vi "Detect change of parameters.vi"(10 "AOL_Globals":T1={"Imaging Protocol"=enum."AOL Z-Stack", "Number of POI"=0, "Number of Miniscans"=0, "Number of Trials"=0, "Number of Cycles "=0, "# Averaged Frames"=0, "Laser power (%)"=0, "Pockels"=0.0, "Acquisition Length (sec)"=0.0, "Fill time (us)"=0.0, "POI Dwell time (us)"=0.0, "Miniscan Dwell time per pixel (us)"=0.0, "PMT 1"=0.0, "PMT 2"=0.0, "Back Apperture"=0.0, "Frame Size"=0, "Center Frequency"=0.0, "Field of View"=0.0, "DwellTime (us)"=0.0, "Wavelength (nm)"=0.0, "Zoom"=0.0, "AOL Z"=0.0, "AOL Mode"=enum."Raster", "GridXY"=0.0, "GridZ"=0.0, "TriggerPeriod (sec)"=0.0, "Number of Pixels in Miniscan"=0, "Experiment folder path"=path "", "X centre"=0.0, "Y centre"=0.0, "Angle (degrees)"=0.0, "Plane Mode"=0, "Threshold"=[], "Regenerate Chirps"=FALSE, "Rectangle ROI length (pixels)"=0, "Rectangle ROI height (pixels)"=0, "AOD fill"=0, "Samples Wait after Trigger"=0, "StartUp Delay"=0, "Slip Cycle"=163840, "Add Cycle"=FALSE} {"Plane Mode" items=["XY Plane"]; "Frame Size" items=["100X100"=100, "128X128"=128, "200X200"=200, "256X256"=256, "512X512"=512, "1024x1024"=1024, "2048x2048"=2048]; "Back Apperture" format="%#.6g"; "Pockels" format="%#.6g"; "PMT 2" format="%#.6g"; "PMT 1" format="%#.6g"; "Angle (degrees)" format="%#.6g"; "POI Dwell time (us)" format="%#.6g"}, 11 "ZStack":cluster{"Zstart":dbl, "Zstop":dbl, "Zstep":dbl}) -> (3 "Setup has changed":bool)   [LabVIEW 2013]
uses:
  Typedefs/Controls/AOL_Globals.ctl
  Typedefs/Imaging Protocols enum.ctl
  Typedefs/Frame Size.ctl
  Typedefs/AOL modes.ctl
  Typedefs/Plane Mode.ctl
  Typedefs/Chirps regen checked params.ctl
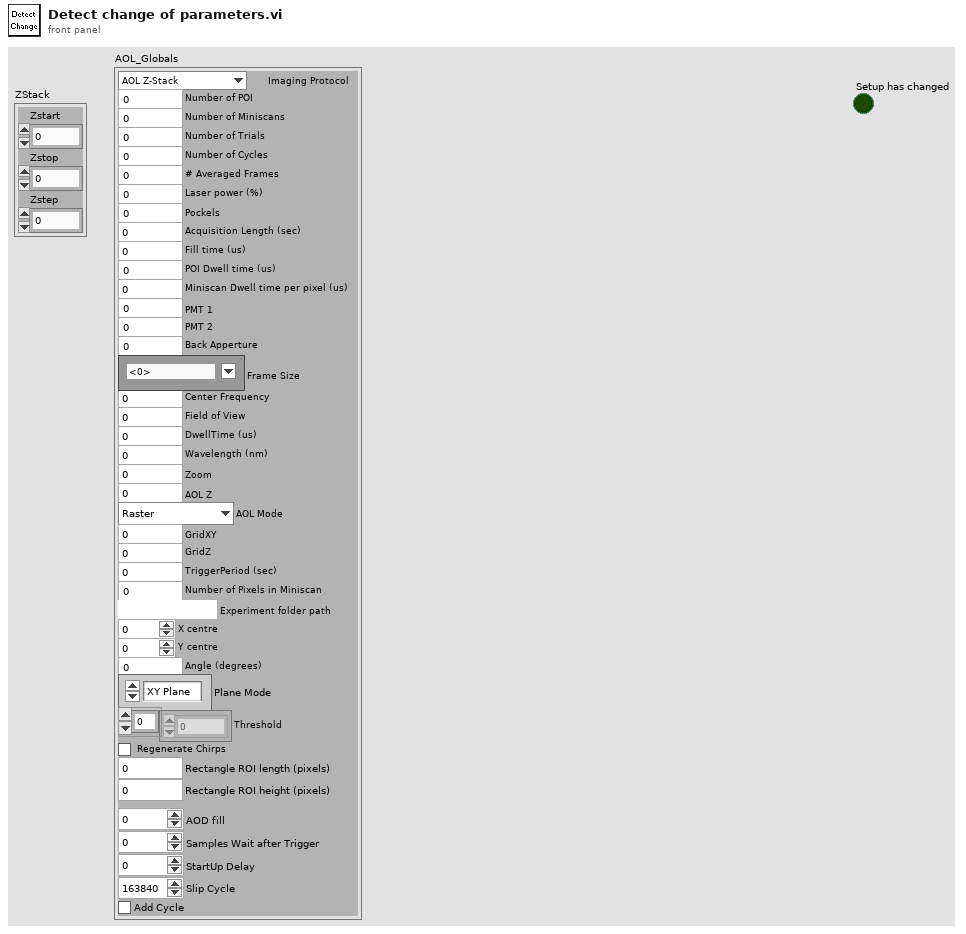
[diagram p1: front panel]
types:
  T1 = typedef "AOL_Globals.ctl" = cluster{"Imaging Protocol":T2, "Number of POI":u16, "Number of Miniscans":u16, "Number of Trials":u16, "Number of Cycles ":u64, "# Averaged Frames":u16, "Laser power (%)":u8, "Pockels":dbl, "Acquisition Length (sec)":dbl, "Fill time (us)":dbl, "POI Dwell time (us)":dbl, "Miniscan Dwell time per pixel (us)":dbl, "PMT 1":dbl, "PMT 2":dbl, "Back Apperture":dbl, "Frame Size":T3, "Center Frequency":dbl, "Field of View":dbl, "DwellTime (us)":dbl, "Wavelength (nm)":dbl, "Zoom":dbl, "AOL Z":dbl, "AOL Mode":T4, "GridXY":dbl, "GridZ":dbl, "TriggerPeriod (sec)":dbl, "Number of Pixels in Miniscan":u16, "Experiment folder path":path, "X centre":dbl, "Y centre":dbl, "Angle (degrees)":dbl, "Plane Mode":T5, "Threshold":u16[], "Regenerate Chirps":bool, "Rectangle ROI length (pixels)":u16, "Rectangle ROI height (pixels)":u16, "AOD fill":u16, "Samples Wait after Trigger":u16, "StartUp Delay":i32, "Slip Cycle":u32, "Add Cycle":bool}
  T2 = typedef "Imaging Protocols enum.ctl" = enum16{"AOL Z-Stack", "Motor Z Stack", "Functional Acquisition", "Single Plane Acquisition", "Volume Acquisition", "Live Imaging", "Live Plane Imaging", "Live Volume Imaging"}
  T3 = typedef "Frame Size.ctl" = u16
  T4 = typedef "AOL modes.ctl" = enum16{"Raster", "Structural", "Pointing", "Mini Scan", "Alignment"}
  T5 = typedef "Plane Mode.ctl" = u16
  T6 = typedef "Chirps regen checked params.ctl" = cluster{"Laser power (%)":u8, "Field of View":dbl, "Frame Size":T3, "AOL Z":dbl, "DwellTime (us)":dbl, "Zoom":dbl, "Number of POI":u16, "Number of Miniscans":u16, "POI Dwell time (us)":dbl, "Miniscan Dwell time per pixel (us)":dbl, "Number of Pixels in Miniscan":u16, "X centre":dbl, "Y centre":dbl, "Wavelength (nm)":dbl, "Angle (degrees)":dbl, "Plane Mode":T5, "Regenerate Chirps":bool}
  T7 = cluster{"ZStack":cluster{"Zstart":dbl, "Zstop":dbl, "Zstep":dbl}, "Checked parameters":T6}
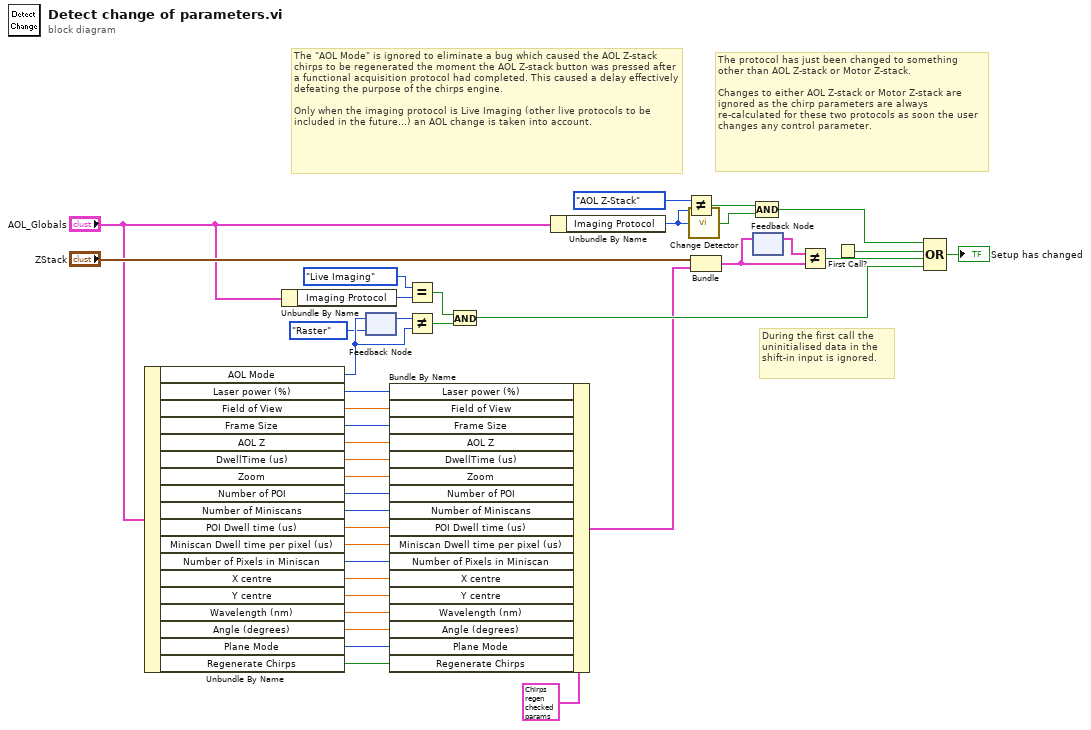
[diagram p0: block diagram]
diagram:
  # "The \"AOL Mode\" is ignored to eliminate a bug which caused the AOL Z-stack chirps to be regenerated the moment the AOL Z-stack button was pressed after a functional acquisition protocol had completed. This caused a delay effectively defeating the purpose of the chirps engine.\n\nOnly when the imaging protocol is Live Imaging (other live protocols to be included in the future...) an AOL change is taken into account."
  # "The protocol has just been changed to something other than AOL Z-stack or Motor Z-stack.\n\nChanges to either AOL Z-stack or Motor Z-stack are ignored as the chirp parameters are always re-calculated for these two protocols as soon the user changes any control parameter."
  # "During the first call the uninitialised data in the shift-in input is ignored."
  n1 = Unbundle By Name("AOL_Globals") -> ("AOL Mode"=w11:T4, "Laser power (%)"=w30:u8, "Field of View"=w29:dbl, "Frame Size"=w28:T3, "AOL Z"=w27:dbl, "DwellTime (us)"=w26:dbl, "Zoom"=w25:dbl, "Number of POI"=w24:u16, "Number of Miniscans"=w23:u16, "POI Dwell time (us)"=w22:dbl, "Miniscan Dwell time per pixel (us)"=w21:dbl, "Number of Pixels in Miniscan"=w20:u16, "X centre"=w19:dbl, "Y centre"=w18:dbl, "Wavelength (nm)"=w17:dbl, "Angle (degrees)"=w16:dbl, "Plane Mode"=w15:T5, "Regenerate Chirps"=w14:bool)
  n2 = Unbundle By Name("AOL_Globals") -> ("Imaging Protocol"=w9:T2)
  n3 = feedback-in #1(w11) -> ()
  n4 = feedback #1(AOL_modes."Raster" ("AOL Mode")) -> (w13:T4)
  n5 = Bundle By Name(cluster=T6 {"Laser power (%)"=0, "Field of View"=0.0, "Frame Size"=0, "AOL Z"=0.0, "DwellTime (us)"=0.0, "Zoom"=0.0, "Number of POI"=0, "Number of Miniscans"=0, "POI Dwell time (us)"=0.0, "Miniscan Dwell time per pixel (us)"=0.0, "Number of Pixels in Miniscan"=0, "X centre"=0.0, "Y centre"=0.0, "Wavelength (nm)"=0.0, "Angle (degrees)"=0.0, "Plane Mode"=0, "Regenerate Chirps"=FALSE} ("Checked parameters"), "Laser power (%)"=w30, "Field of View"=w29, "Frame Size"=w28, "AOL Z"=w27, "DwellTime (us)"=w26, "Zoom"=w25, "Number of POI"=w24, "Number of Miniscans"=w23, "POI Dwell time (us)"=w22, "Miniscan Dwell time per pixel (us)"=w21, "Number of Pixels in Miniscan"=w20, "X centre"=w19, "Y centre"=w18, "Wavelength (nm)"=w17, "Angle (degrees)"=w16, "Plane Mode"=w15, "Regenerate Chirps"=w14) -> (w2:T6)
  n6 = Equal?(x=Imaging_Protocols_enum."Live Imaging", y=w9) -> (x = y?=w8:bool)
  n7 = Not Equal?(x=w13, y=w11) -> (x != y?=w12:bool)
  n8 = And(x=w8, y=w12) -> (x .and. y?=w5:bool)
  n9 = Unbundle By Name("AOL_Globals") -> ("Imaging Protocol"=w34:T2)
  n10 = Not Equal?(x=Imaging_Protocols_enum."AOL Z-Stack", y=w34) -> (x != y?=w35:bool)
  n11 = call <userlib>:"Change Detector.vi"("Value"=w34) -> ("Changed?"=w32:bool)
  n12 = Bundle("ZStack"="ZStack", "Checked parameters"=w2) -> (w6:T7)  [unwired: 1 in]
  n13 = feedback-in #2(w6) -> ()
  n14 = feedback #2() -> (w7:T7)  [unwired: 1 in]
  n15 = Compound Arithmetic op=AND(w35, w32) -> (w31:bool)
  n16 = Not Equal?(x=w7, y=w6) -> (x != y?=w38:bool)
  n17 = First Call?() -> (First Call?: T/F=w39:bool)
  n18 = Compound Arithmetic op=OR(w31, w39, w38, w5) -> (→"Setup has changed":bool)
